vi "Image to Pixmap.vi"(3 "Error":string, 4 "Output Pixmap":u32[][](array[numeric]), 5 "Image":T1={"Image ID"=0, "Channel ID"=-1}) -> (0 "Error":string, 1 "Output Pixmap":u32[][](array[numeric]), 2 "Image":T1={"Image ID"=0, "Channel ID"=-1})   [LabVIEW 2011, in "labvvis.lvlib"]
doc: "Converts a LabVVIS image to a LabVIEW pixmap. This conversion is necessary for LabVIEW to view LabVVIS images."
uses:
  <userlib>/labvvis/labvvis.lvlib
  <userlib>/labvvis/VVIS Image.ctl
  labvvis.framework
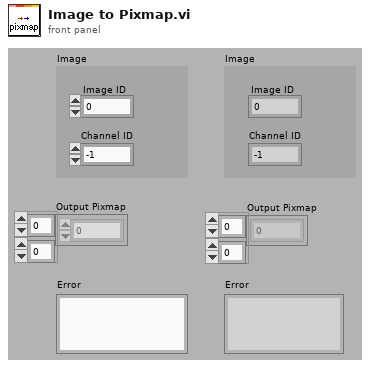
[diagram p1: front panel]
types:
  T1 = typedef "labvvis.lvlib/VVIS Image.ctl" = cluster{"Image ID":i16, "Channel ID":i16}
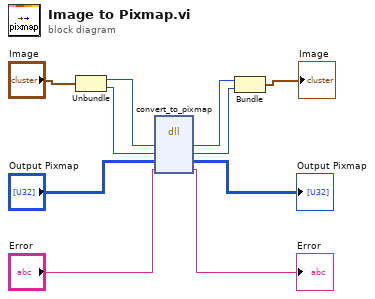
[diagram p0: block diagram]
diagram:
  n1 = Unbundle("Image") -> ("Image ID"=w9:i16, "Channel ID"=w6:i16)
  n2 = dll-call lib="labvvis.framework" fn="convert_to_pixmap"("idnt"=w9, "channel_id"=w6, "pixmap24"="Output Pixmap", "error"="Error") -> ("idnt"=w8:i16, "channel_id"=w2:i16, "pixmap24"=→"Output Pixmap":u32[][], "error"=→"Error":string)  [unwired: 4 in, 2 out]
  n3 = Bundle("idnt"=w8, "channel_id"=w2) -> (→"Image":cluster{"idnt":i16, "channel_id":i16})  [unwired: 1 in]
